vi "Barcode matching.vi"(6 "TFT WORNG SCANE":string="- TFT Barcode Scan Wrong", 8 "TFT BARCODE SCANE":string="- TFT Barcode Scan", 9 "Model":string, 10 "TFT Code":string, 11 "Serial data":string) -> (0 "Error":string, 1 "read buffer":string, 2 "result/trigger":bool, 3 "substring":string, 4 "Read bit":bool)   [LabVIEW 2015]
uses:
  Project Setup/Globle Variable/GR_Servo.vi
  Galobal variable_TI.vi
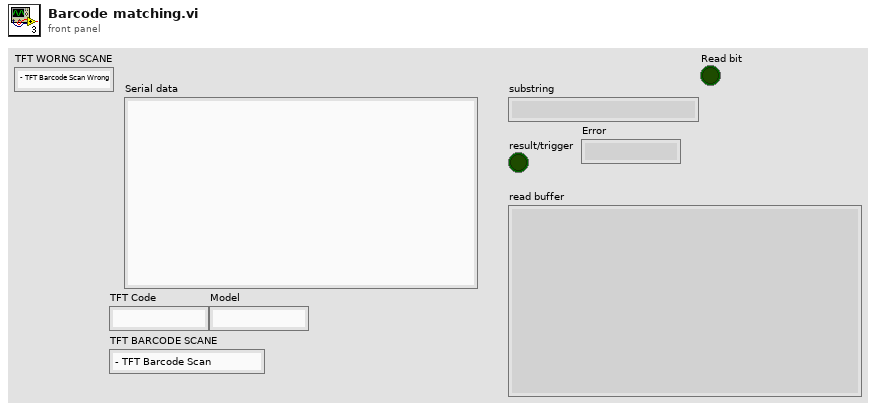
[diagram p1: front panel]
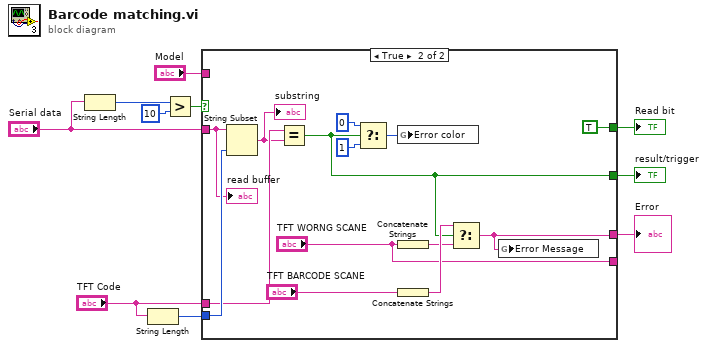
[diagram p0: block diagram]
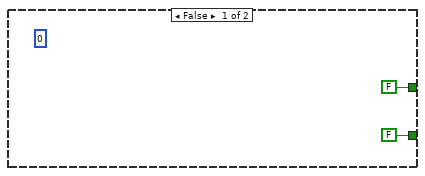
[diagram p2: hidden frame]
diagram:
  n1 = String Length(string="Serial data") -> (length=w6:i32)
  n2 = String Length(string="TFT Code") -> (length=w9:i32)
  n3 = Greater?(x=w6, y=10) -> (0:w8:bool)
  n4 = case shown="True" w8 {
    tunnel: "Serial data" -> [_ w16]
    tunnel: "TFT Code" -> [_ w25]
    tunnel: w9 -> [_ w26]
    tunnel: "Model" -> [_ _]
    tunnel: [FALSE w14] -> w2
    tunnel: [_ "TFT WORNG SCANE"] -> _
    tunnel: [_ w15] -> w3
    tunnel: [FALSE TRUE] -> w1
    frame False {
      (unwired) 0 ("f")
    }
    frame True {
      n5 = String Subset(string=w16, length (rest)=w26) -> (substring=w24:string)  [unwired: 1 in]
      "substring" <- w24
      n6 = Equal?(x=w25, y=w24) -> (x = y?=w14:bool)
      n7 = Select(t=u32 0, s=w14, f=u32 1) -> (s? t:f=w17:u32)
      n8 = global write "Galobal variable_TI.vi" "Error color"(w17) -> ()
      n9 = Concatenate Strings("TFT WORNG SCANE") -> (w19:string)
      n10 = Concatenate Strings("TFT BARCODE SCANE") -> (w20:string)
      n11 = Select(t=w20, s=w14, f=w19) -> (s? t:f=w15:string)
      n12 = global write "GR_Servo.vi" "Error Message"(w15) -> ()
      "read buffer" <- w16
    }
  }
  "Error" <- w3
  "result/trigger" <- w2
  "Read bit" <- w1
